vi "Async Child.vi"(4 "UID":string, 7 "Actor in":refnum<class "Actor.lvclass">, 9 "Mid Actors":refnum<class "Actor.lvclass">[](array[class])) -> (0 "Error out":errorcluster, 5 "Actor out":refnum<class "Actor.lvclass">)   [LabVIEW 2020, in "jettl.lvlib"]
uses:
  jettl.lvlib
  Actor/Actor.lvclass
  Attributes Metadata/Attributes Metadata.lvclass
  Transport/Transport.lvclass
  Attributes/Attributes.lvclass
  Msg/Msg.lvclass
  Base Attributes/Base Attributes.lvlib
  Msgs.ctl
  Attributes.ctl
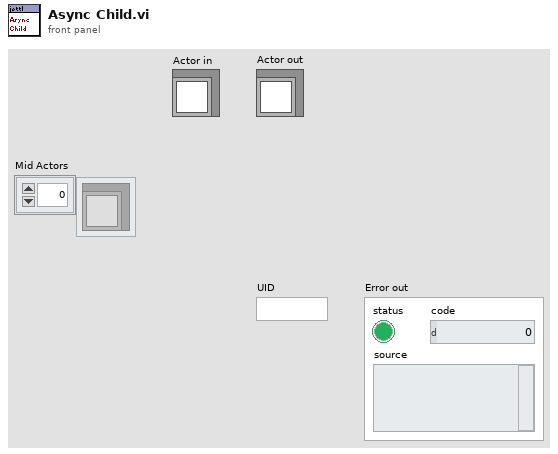
[diagram p1: front panel]
types:
  T1 = typedef "jettl.lvlib/Attributes.ctl" = cluster{"Attributes Metadata":refnum<class "Attributes Metadata.lvclass">, "Unified Msgs":T2, "Edge Actors":refnum<class "Actor.lvclass">[], "Core Actors":refnum<class "Actor.lvclass">[], "Parent Attributes":refnum<class "Attributes.lvclass">, "Root":bool, "UID":string, "Transport":refnum<class "Transport.lvclass">, "VI Ref":refnum<vi>, "Actors":refnum<class "Actor.lvclass">[]}
  T2 = typedef "jettl.lvlib/Msgs.ctl" = set{refnum<class "Msg.lvclass">}
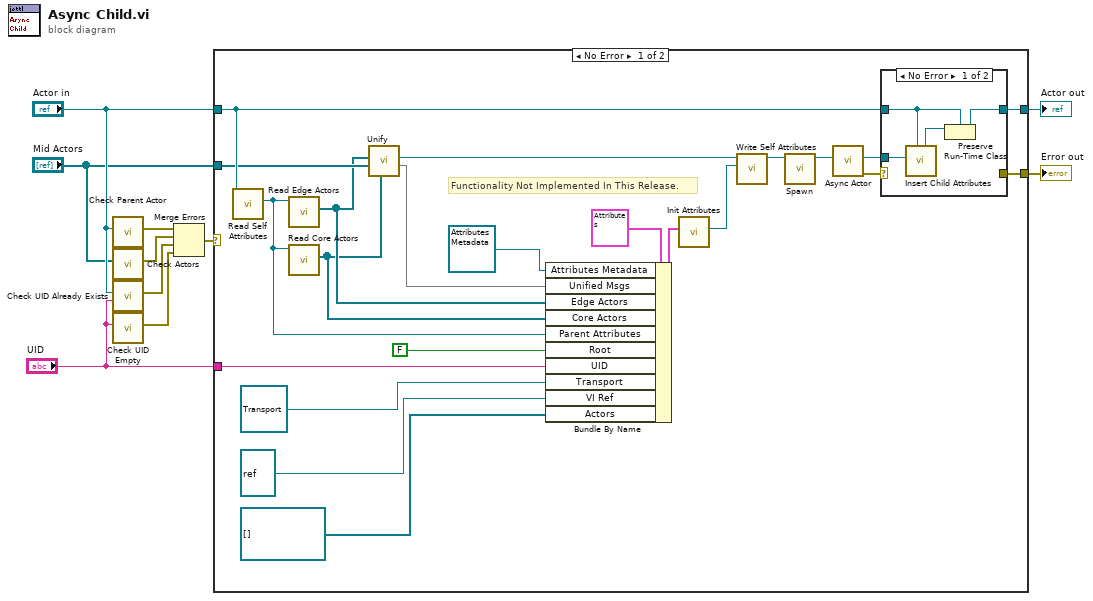
[diagram p0: block diagram]
diagram:
  n1 = call "Check Parent Actor.vi"("Actor"="Actor in") -> ("Error"=w8:errorcluster)  [unwired: 10 in]
  n2 = call "Check Actors.vi"("Actors"="Mid Actors") -> ("Error"=w1:errorcluster)  [unwired: 10 in]
  n3 = call "Check UID Already Exists.vi"("UID"="UID", "Actor"="Actor in") -> ("Error"=w6:errorcluster)  [unwired: 9 in]
  n4 = call "Check UID Empty.vi"("UID"="UID") -> ("Error"=w5:errorcluster)  [unwired: 10 in]
  n5 = Merge Errors(w8, w1, w6, w5) -> (w7:errorcluster)
  n6 = case shown="No Error" w7 {
    selector: w7 -> [_ w39]
    tunnel: "Actor in" -> [w29 w40]
    tunnel: [w32 w39] -> w10
    tunnel: [w31 w40] -> w9
    tunnel: "UID" -> [w24 _]
    tunnel: "Mid Actors" -> [w16 _]
    frame No Error {
      # "Functionality Not Implemented In This Release."
      n7 = call-dynamic "Read Self Attributes.vi"("Actor in"=w29) -> ("Self Attributes"=w17:refnum<class "Attributes.lvclass">)  [unwired: 10 in]
      n8 = call-dynamic "Read Edge Actors.vi"("Attributes in"=w17) -> ("Edge Actors"=w15:refnum<class "Actor.lvclass">[])  [unwired: 10 in]
      n9 = call-dynamic "Read Core Actors.vi"("Attributes in"=w17) -> ("Core Actors"=w14:refnum<class "Actor.lvclass">[])  [unwired: 10 in]
      n10 = call "Unify.vi"("Core Actors"=w14, "Mid Actors"=w16, "Edge Actors"=w15) -> ("Unified Msgs"=w13:T2, "Unified Actor"=w12:refnum<class "Actor.lvclass">)  [unwired: 7 in]
      n11 = Bundle By Name(cluster=T1 {"Attributes Metadata"=refnum, "Unified Msgs"={}, "Edge Actors"=[], "Core Actors"=[], "Parent Attributes"=refnum, "Root"=FALSE, "UID"="", "Transport"=refnum, "VI Ref"=refnum, "Actors"=[]} ("Attributes"), "Attributes Metadata"=refnum<class "Attributes Metadata.lvclass"> refnum, "Unified Msgs"=w13, "Edge Actors"=w15, "Core Actors"=w14, "Parent Attributes"=w17, "Root"=FALSE, "UID"=w24, "Transport"=refnum<class "Transport.lvclass"> refnum, "VI Ref"=refnum<vi> refnum ("Actor Ref"), "Actors"=refnum<class "Actor.lvclass">[] []) -> (w22:T1)
      n12 = call "Init Attributes.vi"("Attributes"=w22) -> ("Attributes"=w30:refnum<class "Attributes.lvclass">)  [unwired: 10 in]
      n13 = call-dynamic "Write Self Attributes.vi"("Self Attributes"=w30, "Actor in"=w12) -> ("Actor out"=w21:refnum<class "Actor.lvclass">)  [unwired: 9 in]
      n14 = call-dynamic "Spawn.vi"("Actor in"=w21) -> ("Actor out"=w20:refnum<class "Actor.lvclass">)  [unwired: 10 in]
      n15 = call "Async Actor.vi"("Unified Actor"=w20) -> ("Error out"=w18:errorcluster, "Child Attributes"=w19:refnum<class "Attributes.lvclass">)  [unwired: 9 in]
      n16 = case shown="No Error" w18 {
        selector: w18 -> [_ w37]
        tunnel: w29 -> [w33 w38]
        tunnel: [w34 w38] -> w31
        tunnel: w19 -> [w36 _]
        tunnel: [_ w37] -> w32
        frame No Error {
          n17 = call "Insert Child Attributes.vi"("Actor in"=w33, "Child Attributes"=w36) -> ("Actor out"=w35:refnum<class "Actor.lvclass">)  [unwired: 9 in]
          n18 = Preserve Run-Time Class(object in=w35, 2:w33) -> (object out=w34:refnum<class "Actor.lvclass">)  [unwired: 1 in, 1 out]
        }
        frame Error {
        }
      }
    }
    frame Error {
    }
  }
  "Actor out" <- w9
  "Error out" <- w10
